vi "Send VHDI-recieveCalibrationStatus.vi"(7 "Message Priority (Normal)":T5=enum."Normal", 8 "error in (no error)":errorcluster, 10 "Calibration Status":T1={"Calib Status"={"Short"=FALSE, "Open"=FALSE, "Load"=FALSE, "Through"=FALSE}, "Calibrated?"=FALSE, "Permativity?"=FALSE, "Progress"={"Progress"=FALSE, "current"=enum."Short", "samples to get"=0}}, 11 "Message Enqueuer":refnum<class "Message Enqueuer.lvclass">) -> (0 "error out":errorcluster, 3 "Message Enqueuer out":refnum<class "Message Enqueuer.lvclass">)   [LabVIEW 2020, in "VDHI-VNA_data_handler_interface.lvlib" / "VHDI-recieveCalibrationStatus Msg.lvclass"]
doc: "This VI sends the message to an actor."
uses:
  VHDI-recieveCalibrationStatus Msg.lvclass
  <vilib>/ActorFramework/Message Enqueuer/Message Enqueuer.lvclass
  <vilib>/ActorFramework/Message Enqueuer/Message Priority.ctl
  VDH-VNA_data_handler/VDH-VNA_data_handler/VDH-calibration_status.ctl
  VDH-VNA_data_handler/VDH-VNA_data_handler/VDH-SOLT_calib_Status.ctl
  VDH-VNA_data_handler/VDH-VNA_data_handler/VDH-Calibration_prosess.ctl
  VDH-VNA_data_handler/VDH-VNA_data_handler/VDH-Calibration_enum.ctl
  C:/Program Files (x86)/National Instruments/LabVIEW 2020/vi.lib/ActorFramework/Message/Message.lvclass
  VHDI-recieveCalibrationStatus Msg.lvclass/VHDI-recieveCalibrationStatus Msg.ctl
  <vilib>/ActorFramework/Message Enqueuer/Message Enqueuer.lvclass/Message Enqueuer.ctl
  <vilib>/ActorFramework/Message Priority Queue/Priority Enqueue.vi
  VDH-VNA_data_handler/VDH-VNA_data_handler/VDH-VNA_data_handler.lvclass
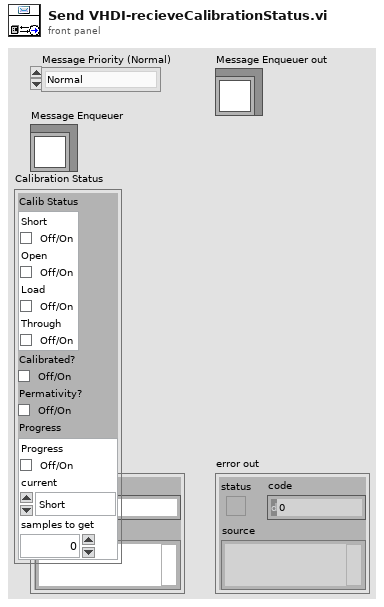
[diagram p1: front panel]
types:
  T1 = typedef "VDH-VNA_data_handler.lvlib/VDH-VNA_data_handler.lvclass/VDH-calibration_status.ctl" = cluster{"Calib Status":T2, "Calibrated?":bool, "Permativity?":bool, "Progress":T3}
  T2 = typedef "VDH-VNA_data_handler.lvlib/VDH-VNA_data_handler.lvclass/VDH-SOLT_calib_Status.ctl" = cluster{"Short":bool, "Open":bool, "Load":bool, "Through":bool}
  T3 = typedef "VDH-VNA_data_handler.lvlib/VDH-VNA_data_handler.lvclass/VDH-Calibration_prosess.ctl" = cluster{"Progress":bool, "current":T4, "samples to get":u8}
  T4 = typedef "VDH-VNA_data_handler.lvlib/VDH-VNA_data_handler.lvclass/VDH-Calibration_enum.ctl" = enum16{"Non", "Short", "Open", "Load", "Through", "Permativity"}
  T5 = typedef "Actor Framework.lvlib/Message Enqueuer.lvclass/Message Priority.ctl" = enum16{"Low", "Normal", "High"}
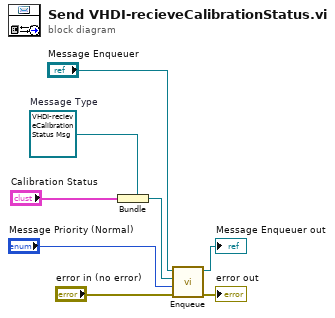
[diagram p0: block diagram]
diagram:
  w5 = refnum<class "VHDI-recieveCalibrationStatus Msg.lvclass"> refnum  # Message Type
  n1 = Bundle(cluster=w5, "Calibration Status") -> (w4:refnum<class "VHDI-recieveCalibrationStatus Msg.lvclass">)
  n2 = call <vilib>:"Enqueue.vi"("error in (no error)"="error in (no error)", "Message Priority (Normal)"="Message Priority (Normal)", "Message"=w4, "Message Enqueuer in"="Message Enqueuer") -> ("error out"=→"error out":errorcluster, "Message Enqueuer out"=→"Message Enqueuer out":refnum<class "Message Enqueuer.lvclass">)  [unwired: 6 in]
